vi "path check.vi"(6 "Base Path":path, 8 "error in (no error)":errorcluster caption="错误输入（无错误）", 9 "Station":string, 10 "Patr Type":string, 11 "Sequence Path":path) -> (0 "error out":errorcluster, 2 "out path":path[](array[path]))   [LabVIEW 2018]
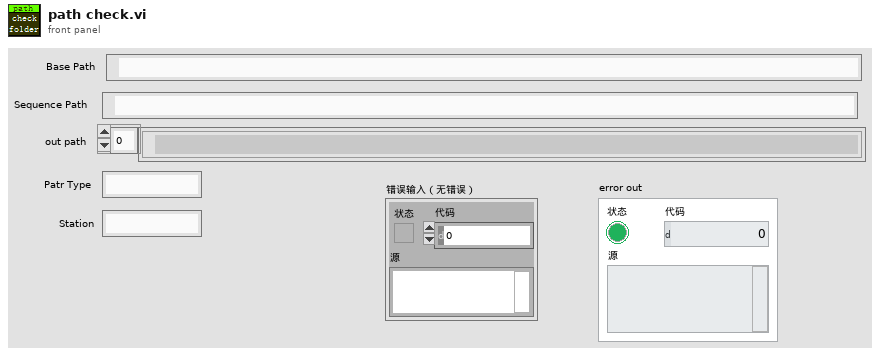
[diagram p1: front panel]
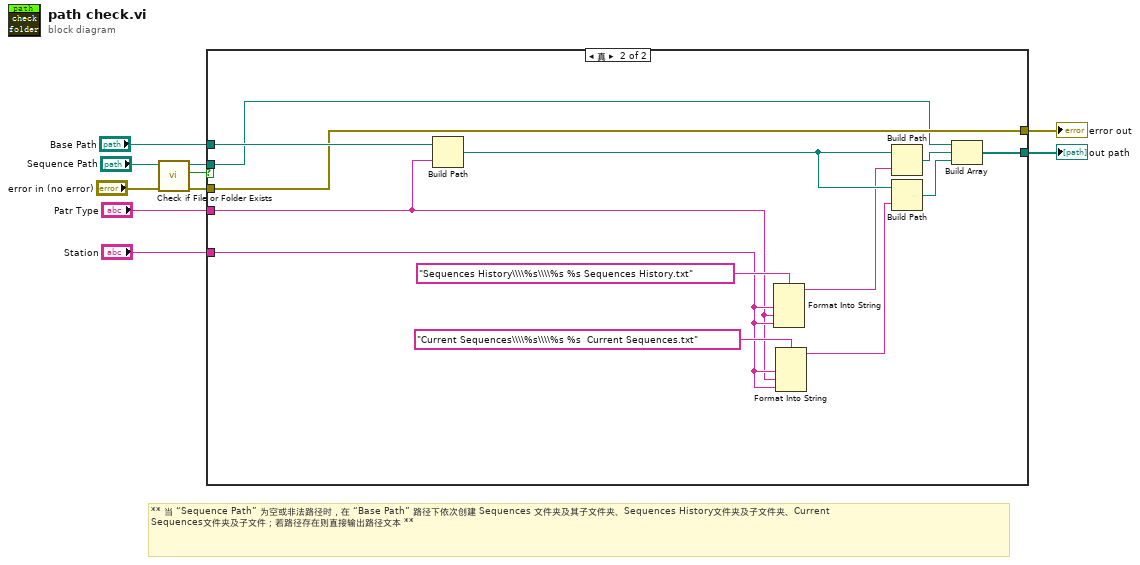
[diagram p0: block diagram]
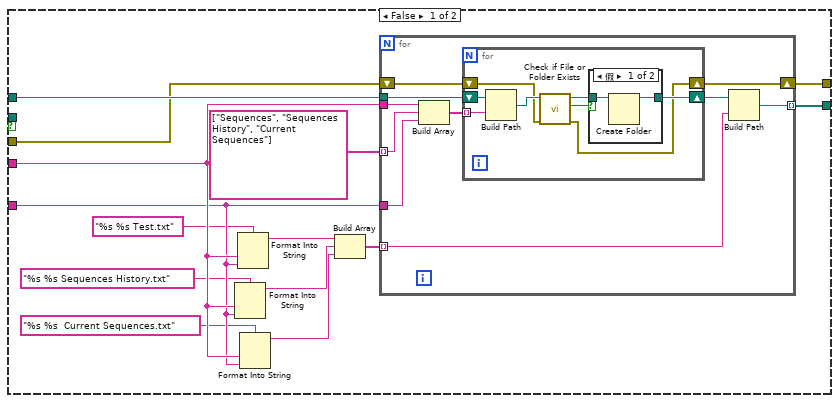
[diagram p2: hidden frame]
diagram:
  # "** 当 “Sequence Path” 为空或非法路径时，在 “Base Path” 路径下依次创建 Sequences 文件夹及其子文件夹、Sequences History文件夹及子文件夹、Current Sequences文件夹及子文件；若路径存在则直接输出路径文本 **"
  n1 = call <vilib>:"Check if File or Folder Exists.vi"("error in (no error)"="error in (no error)", "path"="Sequence Path") -> ("error out"=w5:errorcluster, "file or folder exists?"=w9:bool, "dup path"=w8:path)  [unwired: 7 in]
  n2 = case shown="真" w9 {
    tunnel: w8 -> [_ w46]
    tunnel: "Base Path" -> [w24 w58]
    tunnel: "Patr Type" -> [w17 w50]
    tunnel: "Station" -> [w16 w51]
    tunnel: [w21 w56] -> w6
    tunnel: w5 -> [w12 w47]
    tunnel: [w11 w47] -> w2
    frame False {
      n3 = Format Into String(format string="%s %s Sequences History.txt" ("name or relative path"), w17, w16) -> (resulting string=w19:string)  [unwired: 2 in, 1 out]
      n4 = Format Into String(format string="%s %s Test.txt" ("格式字符串"), w17, w16) -> (resulting string=w20:string)  [unwired: 2 in, 1 out]
      n5 = Format Into String(format string="%s %s  Current Sequences.txt" ("name or relative path"), w17, w16) -> (resulting string=w18:string)  [unwired: 2 in, 1 out]
      n6 = Build Array(w20, w19, w18) -> (w22:string[])
      n7 = for {
        tunnel: w24 -> [w34]
        tunnel: w17 -> [w33]
        tunnel: string[] ["Sequences", "Sequences History", "Current Sequences"] -> [w31] mode=indexing
        tunnel: w16 -> [w30]
        tunnel: w22 -> [w28] mode=indexing
        tunnel: [w27] -> w21 mode=indexing
        shift-right: [w25] -> w11
        shift-left: w12 -> [w26]
        n8 = Build Array(w33, w31, w30) -> (w32:string[])
        n9 = for {
          tunnel: w32 -> [w38] mode=indexing
          shift-right: [w40] -> w29
          shift-left: w34 -> [w39]
          shift-right: [w35] -> w25
          shift-left: w26 -> [w36]
          n10 = Build Path(base path=w39, name or relative path=w38) -> (appended path=w37:path)
          n11 = call <vilib>:"Check if File or Folder Exists.vi"("error in (no error)"=w36, "path"=w37) -> ("error out"=w35:errorcluster, "file or folder exists?"=w42:bool, "dup path"=w41:path)  [unwired: 7 in]
          n12 = case shown="假" w42 {
            tunnel: w41 -> [w44 w45]
            tunnel: [w43 w45] -> w40
            frame False {
              n13 = Create Folder(path (use dialog)=w44) -> (created path=w43:path)  [unwired: 2 in, 2 out]
            }
            frame True {
            }
          }
        }
        n14 = Build Path(base path=w29, name or relative path=w28) -> (appended path=w27:path)
      }
    }
    frame True {
      n15 = Build Path(base path=w58, name or relative path=w50) -> (appended path=w57:path)
      n16 = Format Into String(format string="Sequences History\\\\%s\\\\%s %s Sequences History.txt" ("name or relative path"), w51, w50, w51) -> (resulting string=w49:string)  [unwired: 2 in, 1 out]
      n17 = Format Into String(format string="Current Sequences\\\\%s\\\\%s %s  Current Sequences.txt" ("name or relative path"), w51, w50, w51) -> (resulting string=w48:string)  [unwired: 2 in, 1 out]
      n18 = Build Path(base path=w57, name or relative path=w49) -> (appended path=w55:path)
      n19 = Build Path(base path=w57, name or relative path=w48) -> (appended path=w54:path)
      n20 = Build Array(w46, w55, w54) -> (w56:path[])
    }
  }
  "out path" <- w6
  "error out" <- w2
